vi "Number show.vi"(2 "x":i32=8, 7 "Numeric":u32) -> (8 "Number Array":u16[](array[ring]))   [LabVIEW 2010]
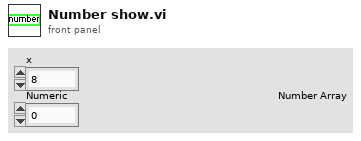
[diagram p1: front panel]
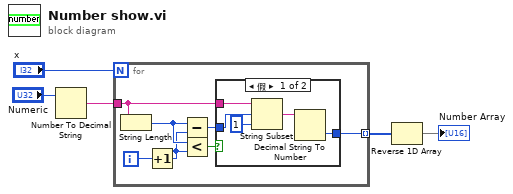
[diagram p0: block diagram]
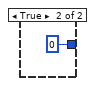
[diagram p2: hidden frame]
diagram:
  n1 = Number To Decimal String(number="Numeric") -> (decimal integer string=w4:string)  [unwired: 1 in]
  n2 = for {
    N: "x" -> [_]
    tunnel: w4 -> [w11]
    tunnel: [w12] -> w2 mode=indexing
    i -> [w9]
    n3 = String Length(string=w11) -> (length=w8:i32)
    n4 = Increment(x=w9) -> (x+1=w6:i32)
    n5 = Subtract(x=w8, y=w6) -> (x-y=w10:i32)
    n6 = Less?(x=w8, y=w6) -> (x < y?=w7:bool)
    n7 = case shown="假" w7 {
      tunnel: [w15 0] -> w12
      tunnel: w11 -> [w14 _]
      tunnel: w10 -> [w13 _]
      frame False {
        n8 = String Subset(string=w14, offset (0)=w13, length (rest)=1 ("length (rest)")) -> (substring=w16:string)
        n9 = Decimal String To Number(string=w16) -> (number=w15:i32)  [unwired: 2 in, 1 out]
      }
      frame True {
      }
    }
  }
  n10 = Reverse 1D Array(array=w2) -> (reversed array=→"Number Array":i32[])
